vi "FTW-Request-Serialize.vi"(0 "Request Header":string, 5 "Request Body":string, 11 "error in":errorcluster) -> (4 "Request":string, 15 "error out":errorcluster)   [LabVIEW 2013, in "FTW-Request.lvclass"]
uses:
  FTW-Request.lvclass
  json/FTW-JSON.lvclass
panel:
  # "Inputs"
  # "Outputs"
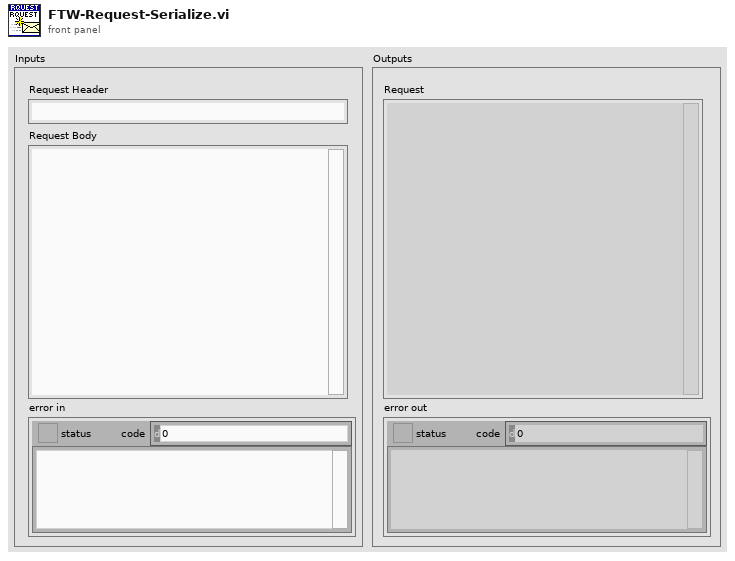
[diagram p1: front panel]
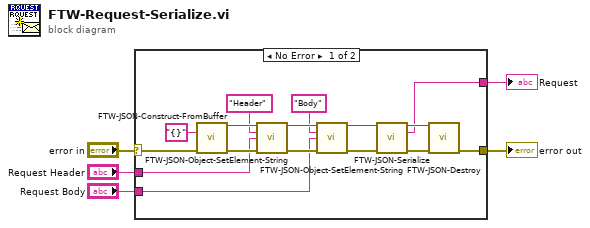
[diagram p0: block diagram]
diagram:
  n1 = case shown="No Error" "error in" {
    selector: "error in" -> [w6 w22]
    tunnel: [w10 w22] -> w5
    tunnel: [w9 _] -> w4
    tunnel: "Request Header" -> [w8 _]
    tunnel: "Request Body" -> [w7 _]
    frame No Error {
      n2 = call "FTW-JSON-Construct-FromBuffer.vi"("JSON String (UTF-8)"="{}", "error in"=w6) -> ("JSON Object"=w20:refnum<class "FTW-JSON.lvclass">, "error out"=w17:errorcluster)  [unwired: 12 in]
      n3 = call "FTW-JSON-Object-SetElement-String.vi"("JSON Object"=w20, "Key"="Header", "Value"=w8, "error in"=w17) -> ("JSON Object out"=w19:refnum<class "FTW-JSON.lvclass">, "error out"=w16:errorcluster)  [unwired: 10 in]
      n4 = call "FTW-JSON-Object-SetElement-String.vi"("JSON Object"=w19, "Key"="Body", "Value"=w7, "error in"=w16) -> ("JSON Object out"=w18:refnum<class "FTW-JSON.lvclass">, "error out"=w15:errorcluster)  [unwired: 10 in]
      n5 = call "FTW-JSON-Serialize.vi"("JSON Object"=w18, "error in"=w15) -> ("JSON Object out"=w13:refnum<class "FTW-JSON.lvclass">, "JSON String (UTF-8)"=w9:string, "error out"=w14:errorcluster)  [unwired: 11 in]
      n6 = call "FTW-JSON-Destroy.vi"("JSON Object"=w13, "error in"=w14) -> ("error out"=w10:errorcluster)  [unwired: 13 in]
    }
    frame Error {
    }
  }
  "error out" <- w5
  "Request" <- w4
